vi "uniqueFile.vi"(11 "PathIn":path=path "C:/Users/cnc/Desktop/junk.csv") -> (3 "PathOut":path)   [LabVIEW 2019]
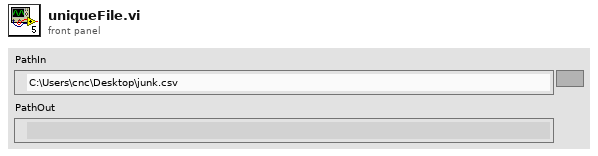
[diagram p1: front panel]
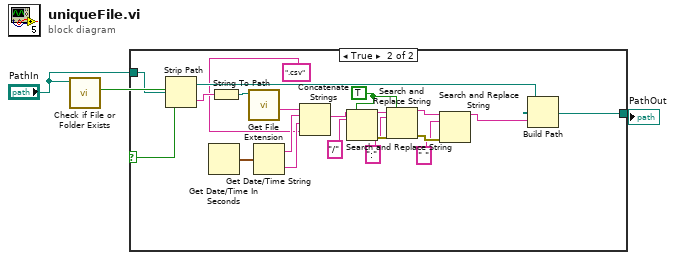
[diagram p0: block diagram]
diagram:
  n1 = call <vilib>:"Check if File or Folder Exists.vi"("path"="PathIn") -> ("file or folder exists?"=w3:bool)  [unwired: 8 in, 2 out]
  n2 = case shown="True" w3 {
    tunnel: "PathIn" -> [w4 w24]
    tunnel: [w4 w14] -> w1
    frame False {
    }
    frame True {
      w10 = TRUE
      n3 = Strip Path(path=w24) -> (stripped path=w17:path, name=w23:string)
      n4 = Get Date/Time In Seconds() -> (seconds since 1Jan1904=w20:timestamp)
      n5 = String To Path(string=w23) -> (path=w22:path)
      n6 = call <vilib>:"Get File Extension.vi"("file"=w22) -> ("filename without extension"=w21:string)  [unwired: 6 in, 4 out]
      n7 = Get Date/Time String(seconds (now)=w20) -> (date string=w19:string, time string=w18:string)  [unwired: 2 in]
      n8 = Concatenate Strings(w21, w19, w18, ".csv") -> (w15:string)
      n9 = Search and Replace String(replace all?=w10, input string=w15, search string="/") -> (result string=w12:string, error out=w13:errorcluster)  [unwired: 5 in, 2 out]
      n10 = Search and Replace String(replace all?=w10, input string=w12, search string=":", error in=w13) -> (result string=w9:string, error out=w8:errorcluster)  [unwired: 4 in, 2 out]
      n11 = Search and Replace String(input string=w9, search string=" ", error in=w8) -> (result string=w7:string)  [unwired: 5 in, 3 out]
      n12 = Build Path(base path=w17, name or relative path=w7) -> (appended path=w14:path)
    }
  }
  "PathOut" <- w1
